vi "Get Host.vi"(8 "error in (no error)":errorcluster, 11 "URI in":refnum<class "URI.lvclass">) -> (0 "error out":errorcluster, 2 "Host":string, 3 "URI out":refnum<class "URI.lvclass">)   [LabVIEW 2020, in "URI.lvclass"]
uses:
  URI.lvclass
  URI.lvclass/URI.ctl
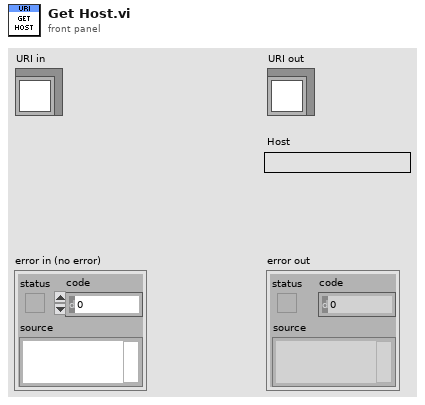
[diagram p1: front panel]
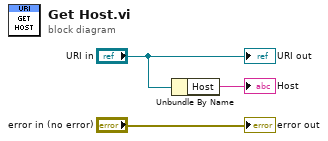
[diagram p0: block diagram]
diagram:
  n1 = Unbundle By Name("URI in") -> ("Host"=→"Host":string)
  "error out" <- "error in (no error)"
  "URI out" <- "URI in"
